vi "Varint Base128 Encoder.vi"(11 "Numeric":u64) -> (3 "Array":u8[](array[numeric]) format="%02x")   [LabVIEW 2023]
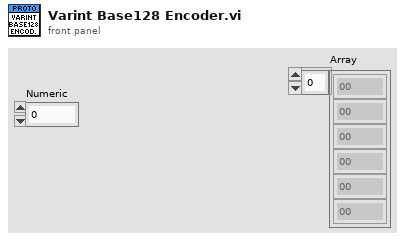
[diagram p1: front panel]
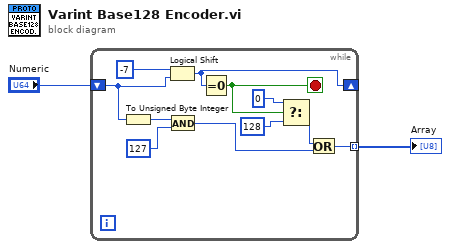
[diagram p0: block diagram]
diagram:
  n1 = while {
    shift-right: [w3] -> _
    shift-left: "Numeric" -> [w4]
    tunnel: [w7] -> w1 mode=indexing
    stop <- w11 stop-if-true
    n2 = To Unsigned Byte Integer(number=w4) -> (unsigned 8bit integer=w6:u8)
    n3 = Logical Shift(y=i16 -7, x=w4) -> (x << y=w3:u64)
    n4 = And(x=w6, y=u8 127) -> (x .and. y?=w8:u8)
    n5 = Equal To 0?(x=w3) -> (x = 0?=w11:bool)
    n6 = Select(t=u8 0, s=w11, f=u8 128) -> (s? t:f=w12:u8)
    n7 = Or(x=w12, y=w8) -> (x .or. y?=w7:u8)
  }
  "Array" <- w1
